vi "ShotCal.vi"() -> ()   [LabVIEW 2015]
uses:
  GlobalVisionVars.vi
  GeneralGlobals.vi
  VisionGlobals.vi
  MotorPositionGlobals.vi
panel:
  in  "Shoot":bool
  in  "enAuto":bool
  out "TargetDistance":dbl
  in  "WinchSetpoint":dbl=4900.0
  in  "TensionerSetpoint":dbl=-90000.0
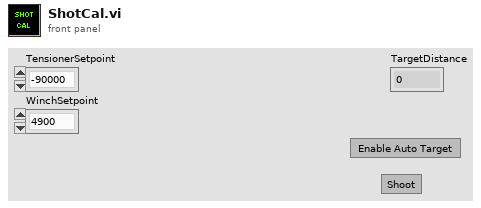
[diagram p1: front panel]
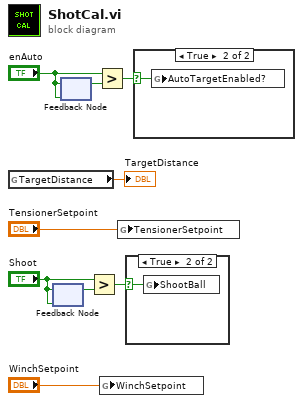
[diagram p0: block diagram]
diagram:
  n1 = global read "GlobalVisionVars.vi" "TargetDistance"() -> (→"TargetDistance":dbl)
  n2 = feedback #1("Shoot") -> (w2:bool)
  n3 = feedback-in #1("Shoot") -> ()
  n4 = feedback-in #2("enAuto") -> ()
  n5 = feedback #2("enAuto") -> (w5:bool)
  n6 = Greater?(x="Shoot", y=w2) -> (0:w3:bool)
  n7 = Greater?(x="enAuto", y=w5) -> (0:w6:bool)
  n8 = global write "MotorPositionGlobals.vi" "WinchSetpoint"("WinchSetpoint") -> ()
  n9 = global write "MotorPositionGlobals.vi" "TensionerSetpoint"("TensionerSetpoint") -> ()
  n10 = case shown="True" w3 {
    selector: w3 -> [_ w10]
    frame False {
    }
    frame True {
      n11 = global write "GeneralGlobals.vi" "ShootBall"(w10) -> ()
    }
  }
  n12 = case shown="True" w6 {
    selector: w6 -> [_ w11]
    frame False {
    }
    frame True {
      n13 = global write "VisionGlobals.vi" "AutoTargetEnabled?"(w11) -> ()
    }
  }
